vi "test_read-nmea-data2.vi"() -> ()   [LabVIEW 2019] (continued)
15:10:14.81\tF9P\t\t\n15:10:14.83\tF9P\t\t\n15:10:14.85\tF9P\t\t\n15:10:14.87\tF9P\t\t\n15:10:14.89\tF9P\t\t\n15:10:14.91\tF9P\t\t\n15:10:14.93\tF9P\t\t\n15:10:14.95\tF9P\t\t\n15:10:14.97\tF9P\t\t\n15:10:14.99\tF9P\t\t\n15:10:15.01\tF9P\t\t\n15:10:15.03\tF9P\t\t\n15:10:15.05\tF9P\t\t\n15:10:15.07\tF9P\t\t\n15:10:15.09\tF9P\t\t\n15:10:15.11\tF9P\t\t\n15:10:15.13\tF9P\t\t\n15:10:15.15\tF9P\t\t\n15:10:15.17\tF9P\t\t\n15:10:15.19\tF9P\t\t\n15:10:15.21\tF9P\t\t\n15:10:15.23\tF9P\t\t\n15:10:15.25\tF9P\t$GNRMC,061017.00,A,3723.57679,N,12656.88354,E,2.166,168.60,250720,,,A,V*08\n\t\n15:10:15.27\tF9P\t$GNVTG,168.60,T,,M,2.166,N,4.012,K,A*2E\n\t\n15:10:15.29\tF9P\t$GNGGA,061017.00,3723.57679,N,12656.88354,E,1,12,0.64,55.0,M,18.5,M,,*75\n\t\n15:10:15.31\tF9P\t$GNGSA,A,3,12,06,19,05,17,09,04,02,,,,,1.19,0.64,1.00,1*0A\n\t\n15:10:15.33\tF9P\t$GNGSA,A,3,85,71,84,,,,,,,,,,1.19,0.64,1.00,2*0F\n\t\n15:10:15.35\tF9P\t$GNGSA,A,3,36,19,11,04,09,12,,,,,,,1.19,0.64,1.00,3*0A\n\t\n15:10:15.37\tF9P\t$GNGSA,A,3,14,11,33,,,,,,,,,,1.19,0.64,1.00,4*0B\n\t\n15:10:15.39\tF9P\t$GPGSV,3,1,09,02,54,318,25,04,19,044,12,05,36,246,25,06,65,046,24,1*68\n\t\n15:10:15.41\tF9P\t$GPGSV,3,2,09,09,45,075,27,12,24,278,17,17,34,153,21,19,53,156,23,1*65\n\t\n15:10:15.43\tF9P\t$GPGSV,3,3,09,25,12,307,,1*5D\n\t\n15:10:15.45\tF9P\t$GPGSV,3,1,09,02,54,318,,04,19,044,,05,36,246,14,06,65,046,16,6*68\n\t\n15:10:15.47\tF9P\t$GPGSV,3,2,09,09,45,075,,12,24,278,,17,34,153,,19,53,156,,6*63\n\t\n15:10:15.49\tF9P\t$GPGSV,3,3,09,25,12,307,,6*5A\n\t\n15:10:15.51\tF9P\t$GLGSV,2,1,08,69,12,031,,70,72,041,,71,51,205,17,72,03,209,,1*74\n\t\n15:10:15.53\tF9P\t$GLGSV,2,2,08,77,01,326,,84,21,121,09,85,70,063,21,86,35,329,,1*7E\n\t\n15:10:15.55\tF9P\t$GLGSV,2,1,08,69,12,031,,70,72,041,,71,51,205,21,72,03,209,,3*73\n\t\n15:10:15.57\tF9P\t$GLGSV,2,2,08,77,01,326,,84,21,121,11,85,70,063,20,86,35,329,,3*74\n\t\n15:10:15.59\tF9P\t$GAGSV,2,1,08,02,09,298,09,04,66,119,25,09,31,193,16,11,71,357,23,7*72\n\t\n15:10:15.61\tF9P\t$GAGSV,2,2,08,12,40,102,15,19,27,045,14,25,09,249,,36,25,308,14,7*7F\n\t\n15:10:15.63\tF9P\t$GAGSV,2,1,08,02,09,298,,04,66,119,23,09,31,193,,11,71,357,19,2*76\n\t\n15:10:15.65\tF9P\t$GAGSV,2,2,08,12,40,102,,19,27,045,,25,09,249,,36,25,308,,2*7E\n\t\n15:10:15.67\tF9P\t$GBGSV,1,1,03,11,50,131,23,14,87,138,20,33,60,219,22,1*4C\n\t\n15:10:15.69\tF9P\t$GBGSV,1,1,03,11,50,131,31,14,87,138,21,33,60,219,,3*4C\n\t\n15:10:15.71\tF9P\t$GNGLL,3723.57679,N,12656.88354,E,061017.00,A,A*7D\n\t\n15:10:15.73\tF9P\t\t\n15:10:15.75\tF9P\t\t\n15:10:15.77\tF9P\t\t\n15:10:15.79\tF9P\t\t\n15:10:15.81\tF9P\t\t\n15:10:15.83\tF9P\t\t\n15:10:15.85\tF9P\t\t\n15:10:15.87\tF9P\t\t\n15:10:15.89\tF9P\t\t\n15:10:15.91\tF9P\t\t\n15:10:15.93\tF9P\t\t\n15:10:15.95\tF9P\t\t\n15:10:15.97\tF9P\t\t\n15:10:15.99\tF9P\t\t\n15:10:16.01\tF9P\t\t\n15:10:16.03\tF9P\t\t\n15:10:16.05\tF9P\t\t\n15:10:16.07\tF9P\t\t\n15:10:16.09\tF9P\t\t\n15:10:16.11\tF9P\t\t\n15:10:16.13\tF9P\t\t\n15:10:16.15\tF9P\t\t\n15:10:16.17\tF9P\t\t\n15:10:16.19\tF9P\t\t\n15:10:16.21\tF9P\t\t\n15:10:16.23\tF9P\t\t\n15:10:16.25\tF9P\t$GNRMC,061018.00,A,3723.57613,N,12656.88385,E,2.313,163.57,250720,,,A,V*08\n\t\n15:10:16.27\tF9P\t$GNVTG,163.57,T,,M,2.313,N,4.284,K,A*2C\n\t\n15:10:16.29\tF9P\t$GNGGA,061018.00,3723.57613,N,12656.88385,E,1,12,0.64,55.5,M,18.5,M,,*7F\n\t\n15:10:16.31\tF9P\t$GNGSA,A,3,12,06,19,05,17,09,04,02,,,,,1.19,0.64,1.00,1*0A\n\t\n15:10:16.33\tF9P\t$GNGSA,A,3,85,71,84,,,,,,,,,,1.19,0.64,1.00,2*0F\n\t\n15:10:16.36\tF9P\t$GNGSA,A,3,36,19,11,04,09,12,,,,,,,1.19,0.64,1.00,3*0A\n\t\n15:10:16.38\tF9P\t$GNGSA,A,3,14,11,33,,,,,,,,,,1.19,0.64,1.00,4*0B\n\t\n15:10:16.40\tF9P\t$GPGSV,3,1,09,02,54,318,25,04,19,044,13,05,36,246,24,06,65,046,25,1*69\n\t\n15:10:16.42\tF9P\t$GPGSV,3,2,09,09,45,075,32,12,24,278,17,17,34,153,23,19,53,156,23,1*63\n\t\n15:10:16.44\tF9P\t$GPGSV,3,3,09,25,12,307,,1*5D\n\t\n15:10:16.46\tF9P\t$GPGSV,3,1,09,02,54,318,,04,19,044,,05,36,246,15,06,65,046,15,6*6A\n\t\n15:10:16.48\tF9P\t$GPGSV,3,2,09,09,45,075,,12,24,278,,17,34,153,,19,53,156,,6*63\n\t\n15:10:16.50\tF9P\t$GPGSV,3,3,09,25,12,307,,6*5A\n\t\n15:10:16.52\tF9P\t$GLGSV,2,1,08,69,12,031,,70,72,041,,71,51,205,16,72,03,209,,1*75\n\t\n15:10:16.54\tF9P\t$GLGSV,2,2,08,77,01,326,,84,21,121,11,85,70,063,21,86,35,329,,1*77\n\t\n15:10:16.56\tF9P\t$GLGSV,2,1,08,69,12,031,,70,72,041,,71,51,205,21,72,03,209,,3*73\n\t\n15:10:16.58\tF9P\t$GLGSV,2,2,08,77,01,326,,84,21,121,09,85,70,063,20,86,35,329,,3*7D\n\t\n15:10:16.60\tF9P\t$GAGSV,2,1,08,02,09,298,10,04,66,119,23,09,31,193,16,11,71,357,24,7*7B\n\t\n15:10:16.62\tF9P\t$GAGSV,2,2,08,12,40,102,16,19,27,045,15,25,09,249,,36,25,308,12,7*7B\n\t\n15:10:16.64\tF9P\t$GAGSV,2,1,08,02,09,298,,04,66,119,,09,31,193,,11,71,357,17,2*79\n\t\n15:10:16.66\tF9P\t$GAGSV,2,2,08,12,40,102,,19,27,045,,25,09,249,,36,25,308,,2*7E\n\t\n15:10:16.68\tF9P\t$GBGSV,1,1,03,11,50,131,22,14,87,138,20,33,60,219,22,1*4D\n\t\n15:10:16.70\tF9P\t$GBGSV,1,1,03,11,50,131,,14,87,138,22,33,60,219,,3*4D\n\t\n15:10:16.72\tF9P\t$GNGLL,3723.57613,N,12656.88385,E,061018.00,A,A*72\n\t\n15:10:16.74\tF9P\t\t\n15:10:16.76\tF9P\t\t\n15:10:16.78\tF9P\t\t\n15:10:16.80\tF9P\t\t\n15:10:16.82\tF9P\t\t\n15:10:16.84\tF9P\t\t\n15:10:16.86\tF9P\t\t\n15:10:16.88\tF9P\t\t\n15:10:16.90\tF9P\t\t\n15:10:16.92\tF9P\t\t\n15:10:16.94\tF9P\t\t\n15:10:16.96\tF9P\t\t\n15:10:16.98\tF9P\t\t\n15:10:17.00\tF9P\t\t\n15:10:17.02\tF9P\t\t\n15:10:17.04\tF9P\t\t\n15:10:17.06\tF9P\t\t\n15:10:17.08\tF9P\t\t\n15:10:17.10\tF9P\t\t\n15:10:17.12\tF9P\t\t\n15:10:17.14\tF9P\t\t\n15:10:17.16\tF9P\t\t\n15:10:17.18\tF9P\t\t\n15:10:17.20\tF9P\t\t\n15:10:17.22\tF9P\t\t\n15:10:17.24\tF9P\t$GNRMC,061019.00,A,3723.57563,N,12656.88365,E,1.827,,250720,,,A,V*14\n\t\n15:10:17.26\tF9P\t$GNVTG,,T,,M,1.827,N,3.383,K,A*3A\n\t\n15:10:17.28\tF9P\t$GNGGA,061019.00,3723.57563,N,12656.88365,E,1,12,0.64,55.5,M,18.5,M,,*74\n\t\n15:10:17.30\tF9P\t$GNGSA,A,3,12,06,19,05,17,09,04,02,,,,,1.19,0.64,1.00,1*0A\n\t\n15:10:17.32\tF9P\t$GNGSA,A,3,85,71,84,,,,,,,,,,1.19,0.64,1.00,2*0F\n\t\n15:10:17.34\tF9P\t$GNGSA,A,3,36,19,11,04,09,12,,,,,,,1.19,0.64,1.00,3*0A\n\t\n15:10:17.36\tF9P\t$GNGSA,A,3,14,11,33,,,,,,,,,,1.19,0.64,1.00,4*0B\n\t\n15:10:17.38\tF9P\t$GPGSV,3,1,09,02,54,318,25,04,19,044,13,05,36,246,25,06,65,046,27,1*6A\n\t\n15:10:17.40\tF9P\t$GPGSV,3,2,09,09,45,075,31,12,24,278,17,17,34,153,22,19,53,156,23,1*61\n\t\n15:10:17.42\tF9P\t$GPGSV,3,3,09,25,12,307,17,1*5B\n\t\n15:10:17.44\tF9P\t$GPGSV,3,1,09,02,54,318,,04,19,044,,05,36,246,16,06,65,046,15,6*69\n\t\n15:10:17.46\tF9P\t$GPGSV,3,2,09,09,45,075,,12,24,278,,17,34,153,,19,53,156,,6*63\n\t\n15:10:17.48\tF9P\t$GPGSV,3,3,09,25,12,307,,6*5A\n\t\n15:10:17.50\tF9P\t$GLGSV,2,1,08,69,12,031,,70,72,041,,71,51,205,17,72,03,209,,1*74\n\t\n15:10:17.52\tF9P\t$GLGSV,2,2,08,77,01,326,,84,21,121,08,85,70,063,19,86,35,329,,1*74\n\t\n15:10:17.54\tF9P\t$GLGSV,2,1,08,69,12,031,,70,72,041,,71,51,205,20,72,03,209,,3*72\n\t\n15:10:17.56\tF9P\t$GLGSV,2,2,08,77,01,326,,84,21,121,11,85,70,063,19,86,35,329,,3*7E\n\t\n15:10:17.58\tF9P\t$GAGSV,2,1,08,02,09,298,12,04,66,119,22,09,31,193,17,11,71,357,23,7*7E\n\t\n15:10:17.60\tF9P\t$GAGSV,2,2,08,12,40,102,15,19,27,045,16,25,09,249,,36,25,308,13,7*7A\n\t\n15:10:17.62\tF9P\t$GAGSV,2,1,08,02,09,298,,04,66,119,,09,31,193,,11,71,357,14,2*7A\n\t\n15:10:17.64\tF9P\t$GAGSV,2,2,08,12,40,102,,19,27,045,,25,09,249,,36,25,308,,2*7E\n\t\n15:10:17.66\tF9P\t$GBGSV,1,1,03,11,50,131,21,14,87,138,19,33,60,219,21,1*47\n\t\n15:10:17.68\tF9P\t$GBGSV,1,1,03,11,50,131,,14,87,138,20,33,60,219,,3*4F\n\t\n15:10:17.70\tF9P\t$GNGLL,3723.57563,N,12656.88365,E,061019.00,A,A*79\n\t\n15:10:17.72\tF9P\t\t\n15:10:17.74\tF9P\t\t\n15:10:17.76\tF9P\t\t\n15:10:17.78\tF9P\t\t\n15:10:17.80\tF9P\t\t\n15:10:17.82\tF9P\t\t\n15:10:17.84\tF9P\t\t\n15:10:17.86\tF9P\t\t\n15:10:17.88\tF9P\t\t\n15:10:17.90\tF9P\t\t\n15:10:17.92\tF9P\t\t\n15:10:17.94\tF9P\t\t\n15:10:17.96\tF9P\t\t\n15:10:17.98\tF9P\t\t\n15:10:18.00\tF9P\t\t\n15:10:18.02\tF9P\t\t\n15:10:18.04\tF9P\t\t\n15:10:18.06\tF9P\t\t\n15:10:18.08\tF9P\t\t\n15:10:18.10\tF9P\t\t\n15:10:18.12\tF9P\t\t\n15:10:18.14\tF9P\t\t\n15:10:18.16\tF9P\t\t\n15:10:18.18\tF9P\t\t\n15:10:18.20\tF9P\t\t\n15:10:18.22\tF9P\t\t\n15:10:18.24\tF9P\t$GNRMC,061020.00,A,3723.57529,N,12656.88348,E,1.000,,250720,,,A,V*12\n\t\n15:10:18.26\tF9P\t$GNVTG,,T,,M,1.000,N,1.853,K,A*33\n\t\n15:10:18.28\tF9P\t$GNGGA,061020.00,3723.57529,N,12656.88348,E,1,12,0.64,56.6,M,18.5,M,,*7F\n\t\n15:10:18.30\tF9P\t$GNGSA,A,3,12,06,19,05,17,09,04,02,,,,,1.19,0.64,1.00,1*0A\n\t\n15:10:18.32\tF9P\t$GNGSA,A,3,85,71,84,,,,,,,,,,1.19,0.64,1.00,2*0F\n\t\n15:10:18.34\tF9P\t$GNGSA,A,3,36,19,11,04,09,12,,,,,,,1.19,0.64,1.00,3*0A\n\t\n15:10:18.36\tF9P\t$GNGSA,A,3,14,11,33,,,,,,,,,,1.19,0.64,1.00,4*0B\n\t\n15:10:18.38\tF9P\t$GPGSV,3,1,09,02,54,318,24,04,19,044,13,05,36,246,23,06,65,046,26,1*6C\n\t\n15:10:18.40\tF9P\t$GPGSV,3,2,09,09,45,075,30,12,24,278,17,17,34,153,22,19,53,156,24,1*67\n\t\n15:10:18.42\tF9P\t$GPGSV,3,3,09,25,12,307,15,1*59\n\t\n15:10:18.44\tF9P\t$GPGSV,3,1,09,02,54,318,,04,19,044,,05,36,246,15,06,65,046,15,6*6A\n\t\n15:10:18.46\tF9P\t$GPGSV,3,2,09,09,45,075,,12,24,278,,17,34,153,,19,53,156,,6*63\n\t\n15:10:18.48\tF9P\t$GPGSV,3,3,09,25,12,307,,6*5A\n\t\n15:10:18.50\tF9P\t$GLGSV,2,1,08,69,12,031,,70,72,041,,71,51,205,17,72,03,209,,1*74\n\t\n15:10:18.52\tF9P\t$GLGSV,2,2,08,77,01,326,,84,21,121,09,85,70,063,18,86,35,329,,1*74\n\t\n15:10:18.54\tF9P\t$GLGSV,2,1,08,69,12,031,,70,72,041,,71,51,205,20,72,03,209,,3*72\n\t\n15:10:18.56\tF9P\t$GLGSV,2,2,08,77,01,326,,84,21,121,08,85,70,063,19,86,35,329,,3*76\n\t\n15:10:18.58\tF9P\t$GAGSV,2,1,08,02,09,298,06,04,66,119,23,09,31,193,18,11,71,357,25,7*73\n\t\n15:10:18.60\tF9P\t$GAGSV,2,2,08,12,40,102,14,19,27,045,16,25,09,249,,36,25,308,14,7*7C\n\t\n15:10:18.62\tF9P\t$GAGSV,2,1,08,02,09,298,,04,66,119,,09,31,193,,11,71,357,14,2*7A\n\t\n15:10:18.64\tF9P\t$GAGSV,2,2,08,12,40,102,,19,27,045,,25,09,249,,36,25,308,,2*7E\n\t\n15:10:18.66\tF9P\t$GBGSV,1,1,03,11,50,131,21,14,87,138,19,33,60,219,21,1*47\n\t\n15:10:18.68\tF9P\t$GBGSV,1,1,03,11,50,131,,14,87,138,22,33,60,219,,3*4D\n\t\n15:10:18.70\tF9P\t$GNGLL,3723.57529,N,12656.88348,E,061020.00,A,A*72\n\t\n15:10:18.72\tF9P\t\t\n15:10:18.74\tF9P\t\t\n15:10:18.76\tF9P\t\t\n15:10:18.78\tF9P\t\t\n15:10:18.80\tF9P\t\t\n15:10:18.82\tF9P\t\t\n15:10:18.84\tF9P\t\t\n15:10:18.86\tF9P\t\t\n15:10:18.88\tF9P\t\t\n15:10:18.90\tF9P\t\t\n15:10:18.92\tF9P\t\t\n15:10:18.94\tF9P\t\t\n15:10:18.96\tF9P\t\t\n15:10:18.98\tF9P\t\t\n15:10:19.00\tF9P\t\t\n15:10:19.02\tF9P\t\t\n15:10:19.04\tF9P\t\t\n15:10:19.06\tF9P\t\t\n15:10:19.08\tF9P\t\t\n15:10:19.10\tF9P\t\t\n15:10:19.12\tF9P\t\t\n15:10:19.14\tF9P\t\t\n15:10:19.16\tF9P\t\t\n15:10:19.18\tF9P\t\t\n15:10:19.20\tF9P\t\t\n15:10:19.22\tF9P\t\t\n15:10:19.24\tF9P\t$GNRMC,061021.00,A,3723.57492,N,12656.88360,E,1.046,,250720,,,A,V*1A\n\t\n15:10:19.26\tF9P\t$GNVTG,,T,,M,1.046,N,1.938,K,A*3D\n\t\n15:10:19.28\tF9P\t$GNGGA,061021.00,3723.57492,N,12656.88360,E,1,12,0.64,57.4,M,18.5,M,,*76\n\t\n15:10:19.30\tF9P\t$GNGSA,A,3,12,06,19,05,17,09,04,02,,,,,1.19,0.64,1.00,1*0A\n\t\n15:10:19.32\tF9P\t$GNGSA,A,3,85,71,84,,,,,,,,,,1.19,0.64,1.00,2*0F\n\t\n15:10:19.34\tF9P\t$GNGSA,A,3,36,19,11,04,09,12,,,,,,,1.19,0.64,1.00,3*0A\n\t\n15:10:19.36\tF9P\t$GNGSA,A,3,14,11,33,,,,,,,,,,1.19,0.64,1.00,4*0B\n\t\n15:10:19.38\tF9P\t$GPGSV,3,1,09,02,54,318,24,04,19,044,12,05,36,246,28,06,65,046,25,1*65\n\t\n15:10:19.40\tF9P\t$GPGSV,3,2,09,09,45,075,23,12,24,278,18,17,34,153,22,19,53,156,25,1*6B\n\t\n15:10:19.42\tF9P\t$GPGSV,3,3,09,25,12,307,14,1*58\n\t\n15:10:19.44\tF9P\t$GPGSV,3,1,09,02,54,318,,04,19,044,,05,36,246,15,06,65,046,14,6*6B\n\t\n15:10:19.46\tF9P\t$GPGSV,3,2,09,09,45,075,,12,24,278,,17,34,153,,19,53,156,,6*63\n\t\n15:10:19.48\tF9P\t$GPGSV,3,3,09,25,12,307,,6*5A\n\t\n15:10:19.50\tF9P\t$GLGSV,2,1,08,69,12,031,,70,72,041,,71,51,205,19,72,03,209,,1*7A\n\t\n15:10:19.52\tF9P\t$GLGSV,2,2,08,77,01,326,,84,20,122,11,85,70,063,20,86,35,329,,1*74\n\t\n15:10:19.54\tF9P\t$GLGSV,2,1,08,69,12,031,,70,72,041,,71,51,205,20,72,03,209,,3*72\n\t\n15:10:19.56\tF9P\t$GLGSV,2,2,08,77,01,326,,84,20,122,10,85,70,063,18,86,35,329,,3*7C\n\t\n15:10:19.58\tF9P\t$GAGSV,2,1,08,02,09,298,09,04,66,119,23,09,31,193,18,11,71,357,24,7*7D\n\t\n15:10:19.60\tF9P\t$GAGSV,2,2,08,12,40,102,14,19,27,045,16,25,09,249,,36,25,308,14,7*7C\n\t\n15:10:19.62\tF9P\t$GAGSV,2,1,08,02,09,298,,04,66,119,,09,31,193,27,11,71,357,15,2*7E\n\t\n15:10:19.64\tF9P\t$GAGSV,2,2,08,12,40,102,,19,27,045,,25,09,249,,36,25,308,,2*7E\n\t\n15:10:19.66\tF9P\t$GBGSV,1,1,03,11,50,131,20,14,87,138,19,33,60,219,21,1*46\n\t\n15:10:19.68\tF9P\t$GBGSV,1,1,03,11,50,131,,14,87,138,22,33,60,219,,3*4D\n\t\n15:10:19.70\tF9P\t$GNGLL,3723.57492,N,12656.88360,E,061021.00,A,A*78\n\t\n15:10:19.72\tF9P\t\t\n15:10:19.74\tF9P\t\t\n15:10:19.76\tF9P\t\t\n15:10:19.78\tF9P\t\t\n15:10:19.80\tF9P\t\t\n15:10:19.82\tF9P\t\t\n15:10:19.84\tF9P\t\t\n15:10:19.86\tF9P\t\t\n15:10:19.88\tF9P\t\t\n15:10:19.90\tF9P\t\t\n15:10:19.92\tF9P\t\t\n15:10:19.94\tF9P\t\t\n15:10:19.96\tF9P\t\t\n15:10:19.98\tF9P\t\t\n15:10:20.00\tF9P\t\t\n15:10:20.02\tF9P\t\t\n15:10:20.04\tF9P\t\t\n15:10:20.06\tF9P\t\t\n15:10:20.08\tF9P\t\t\n15:10:20.10\tF9P\t\t\n15:10:20.12\tF9P\t\t\n15:10:20.14\tF9P\t\t\n15:10:20.16\tF9P\t\t\n15:10:20.18\tF9P\t\t\n15:10:20.20\tF9P\t\t\n15:10:20.22\tF9P\t\t\n15:10:20.24\tF9P\t$GNRMC,061022.00,A,3723.57424,N,12656.88360,E,1.903,,250720,,,A,V*1C\n\t\n15:10:20.26\tF9P\t$GNVTG,,T,,M,1.903,N,3.524,K,A*36\n\t\n15:10:20.28\tF9P\t$GNGGA,061022.00,3723.57424,N,12656.88360,E,1,12,0.64,57.6,M,18.5,M,,*7A\n\t\n15:10:20.30\tF9P\t$GNGSA,A,3,12,06,19,05,17,09,04,02,,,,,1.19,0.64,1.00,1*0A\n\t\n15:10:20.32\tF9P\t$GNGSA,A,3,85,71,84,,,,,,,,,,1.19,0.64,1.00,2*0F\n\t\n15:10:20.34\tF9P\t$GNGSA,A,3,36,19,11,04,09,12,,,,,,,1.19,0.64,1.00,3*0A\n\t\n15:10:20.36\tF9P\t$GNGSA,A,3,14,11,33,,,,,,,,,,1.19,0.64,1.00,4*0B\n\t\n15:10:20.38\tF9P\t$GPGSV,3,1,09,02,54,318,24,04,19,044,12,05,36,246,24,06,65,046,31,1*6C\n\t\n15:10:20.40\tF9P\t$GPGSV,3,2,09,09,45,075,30,12,24,278,19,17,34,153,23,19,53,156,22,1*6E\n\t\n15:10:20.42\tF9P\t$GPGSV,3,3,09,25,12,307,14,1*58\n\t\n15:10:20.44\tF9P\t$GPGSV,3,1,09,02,54,318,,04,19,044,,05,36,246,16,06,65,046,13,6*6F\n\t\n15:10:20.46\tF9P\t$GPGSV,3,2,09,09,45,075,,12,24,278,,17,34,153,,19,53,156,,6*63\n\t\n15:10:20.48\tF9P\t$GPGSV,3,3,09,25,12,307,,6*5A\n\t\n15:10:20.50\tF9P\t$GLGSV,2,1,08,69,12,031,,70,72,041,,71,51,205,20,72,03,209,,1*70\n\t\n15:10:20.52\tF9P\t$GLGSV,2,2,08,77,01,326,,84,20,122,08,85,70,065,20,86,35,329,,1*7A\n\t\n15:10:20.54\tF9P\t$GLGSV,2,1,08,69,12,031,,70,72,041,,71,51,205,20,72,03,209,,3*72\n\t\n15:10:20.56\tF9P\t$GLGSV,2,2,08,77,01,326,,84,20,122,08,85,70,065,19,86,35,329,,3*72\n\t\n15:10:20.58\tF9P\t$GAGSV,2,1,08,02,09,298,08,04,66,119,22,09,31,193,17,11,71,357,24,7*72\n\t\n15:10:20.60\tF9P\t$GAGSV,2,2,08,12,40,102,12,19,27,045,15,25,09,249,,36,25,308,15,7*78\n\t\n15:10:20.62\tF9P\t$GAGSV,2,1,08,02,09,298,,04,66,119,,09,31,193,24,11,71,357,15,2*7D\n\t\n15:10:20.64\tF9P\t$GAGSV,2,2,08,12,40,102,,19,27,045,,25,09,249,,36,25,308,,2*7E\n\t\n15:10:20.66\tF9P\t$GBGSV,1,1,03,11,50,131,20,14,87,138,20,33,60,219,21,1*4C\n\t\n15:10:20.68\tF9P\t$GBGSV,1,1,03,11,50,131,,14,87,138,22,33,60,219,,3*4D\n\t\n15:10:20.70\tF9P\t$GNGLL,3723.57424,N,12656.88360,E,061022.00,A,A*76\n\t\n15:10:20.72\tF9P\t\t\n15:10:20.74\tF9P\t\t\n15:10:20.76\tF9P\t\t\n15:10:20.78\tF9P\t\t\n15:10:20.80\tF9P\t\t\n15:10:20.82\tF9P\t\t\n15:10:20.84\tF9P\t\t\n15:10:20.86\tF9P\t\t\n15:10:20.88\tF9P\t\t\n15:10:20.91\tF9P\t\t\n15:10:20.93\tF9P\t\t\n15:10:20.95\tF9P\t\t\n15:10:20.97\tF9P\t\t\n15:10:20.99\tF9P\t\t\n15:10:21.01\tF9P\t\t\n15:10:21.03\tF9P\t\t\n15:10:21.05\tF9P\t\t\n15:10:21.07\tF9P\t\t\n15:10:21.09\tF9P\t\t\n15:10:21.11\tF9P\t\t\n15:10:21.12\tF9P\t\t\n15:10:21.14\tF9P\t\t\n15:10:21.16\tF9P\t\t\n15:10:21.18\tF9P\t\t\n15:10:21.20\tF9P\t\t\n15:10:21.22\tF9P\t\t\n15:10:21.24\tF9P\t$GNRMC,061023.00,A,3723.57354,N,12656.88377,E,1.992,,250720,,,A,V*13\n\t\n15:10:21.26\tF9P\t$GNVTG,,T,,M,1.992,N,3.689,K,A*3A\n\t\n15:10:21.28\tF9P\t$GNGGA,061023.00,3723.57354,N,12656.88377,E,1,12,0.64,58.0,M,18.5,M,,*74\n\t\n15:10:21.30\tF9P\t$GNGSA,A,3,12,06,19,05,17,09,04,02,,,,,1.19,0.64,1.00,1*0A\n\t\n15:10:21.32\tF9P\t$GNGSA,A,3,85,71,84,,,,,,,,,,1.19,0.64,1.00,2*0F\n\t\n15:10:21.34\tF9P\t$GNGSA,A,3,36,19,11,04,09,12,,,,,,,1.19,0.64,1.00,3*0A\n\t\n15:10:21.36\tF9P\t$GNGSA,A,3,14,11,33,,,,,,,,,,1.19,0.64,1.00,4*0B\n\t\n15:10:21.38\tF9P\t$GPGSV,3,1,09,02,54,318,23,04,19,044,12,05,36,246,24,06,65,046,25,1*6E\n\t\n15:10:21.40\tF9P\t$GPGSV,3,2,09,09,45,075,24,12,24,278,18,17,34,153,22,19,53,156,22,1*6B\n\t\n15:10:21.42\tF9P\t$GPGSV,3,3,09,25,12,307,15,1*59\n\t\n15:10:21.44\tF9P\t$GPGSV,3,1,09,02,54,318,,04,19,044,,05,36,246,17,06,65,046,12,6*6F\n\t\n15:10:21.46\tF9P\t$GPGSV,3,2,09,09,45,075,,12,24,278,,17,34,153,,19,53,156,,6*63\n\t\n15:10:21.48\tF9P\t$GPGSV,3,3,09,25,12,307,,6*5A\n\t\n15:10:21.50\tF9P\t$GLGSV,2,1,08,69,12,031,,70,72,041,,71,51,205,19,72,03,209,,1*7A\n\t\n15:10:21.52\tF9P\t$GLGSV,2,2,08,77,01,326,,84,20,122,08,85,70,065,21,86,36,330,,1*70\n\t\n15:10:21.54\tF9P\t$GLGSV,2,1,08,69,12,031,,70,72,041,,71,51,205,20,72,03,209,,3*72\n\t\n15:10:21.56\tF9P\t$GLGSV,2,2,08,77,01,326,,84,20,122,10,85,70,065,19,86,36,330,,3*70\n\t\n15:10:21.58\tF9P\t$GAGSV,2,1,08,02,09,298,08,04,66,119,22,09,31,193,17,11,71,357,24,7*72\n\t\n15:10:21.60\tF9P\t$GAGSV,2,2,08,12,40,102,10,19,27,045,18,25,09,249,,36,25,308,14,7*76\n\t\n15:10:21.62\tF9P\t$GAGSV,2,1,08,02,09,298,,04,66,119,,09,31,193,21,11,71,357,12,2*7F\n\t\n15:10:21.64\tF9P\t$GAGSV,2,2,08,12,40,102,,19,27,045,,25,09,249,,36,25,308,,2*7E\n\t\n15:10:21.66\tF9P\t$GBGSV,1,1,03,11,50,131,21,14,87,138,20,33,60,219,21,1*4D\n\t\n15:10:21.68\tF9P\t$GBGSV,1,1,03,11,50,131,,14,87,138,21,33,60,219,,3*4E\n\t\n15:10:21.70\tF9P\t$GNGLL,3723.57354,N,12656.88377,E,061023.00,A,A*71\n\t\n15:10:21.72\tF9P\t\t\n15:10:21.74\tF9P\t\t\n15:10:21.76\tF9P\t\t\n15:10:21.78\tF9P\t\t\n15:10:21.80\tF9P\t\t\n15:10:21.82\tF9P\t\t\n15:10:21.84\tF9P\t\t\n15:10:21.86\tF9P\t\t\n15:10:21.88\tF9P\t\t\n15:10:21.90\tF9P\t\t\n15:10:21.92\tF9P\t\t\n15:10:21.94\tF9P\t\t\n15:10:21.96\tF9P\t\t\n15:10:21.98\tF9P\t\t\n15:10:22.00\tF9P\t\t\n15:10:22.02\tF9P\t\t\n15:10:22.04\tF9P\t\t\n15:10:22.06\tF9P\t\t\n15:10:22.08\tF9P\t\t\n15:10:22.10\tF9P\t\t\n15:10:22.12\tF9P\t\t\n15:10:22.14\tF9P\t\t\n15:10:22.16\tF9P\t\t\n15:10:22.18\tF9P\t\t\n15:10:22.20\tF9P\t\t\n15:10:22.22\tF9P\t\t\n15:10:22.24\tF9P\t$GNRMC,061024.00,A,3723.57293,N,12656.88370,E,1.879,,250720,,,A,V*1D\n\t\n15:10:22.26\tF9P\t$GNVTG,,T,,M,1.879,N,3.480,K,A*35\n\t\n15:10:22.28\tF9P\t$GNGGA,061024.00,3723.57293,N,12656.88370,E,1,12,0.65,59.5,M,18.5,M,,*7B\n\t\n15:10:22.30\tF9P\t$GNGSA,A,3,12,06,19,05,17,09,04,02,,,,,1.19,0.65,1.00,1*0B\n\t\n15:10:22.32\tF9P\t$GNGSA,A,3,85,71,84,,,,,,,,,,1.19,0.65,1.00,2*0E\n\t\n15:10:22.34\tF9P\t$GNGSA,A,3,36,19,11,04,09,,,,,,,,1.19,0.65,1.00,3*08\n\t\n15:10:22.36\tF9P\t$GNGSA,A,3,14,11,33,,,,,,,,,,1.19,0.65,1.00,4*0A\n\t\n15:10:22.38\tF9P\t$GPGSV,3,1,09,02,54,318,22,04,19,044,13,05,36,246,25,06,65,046,25,1*6F\n\t\n15:10:22.40\tF9P\t$GPGSV,3,2,09,09,45,075,25,12,24,278,18,17,34,153,22,19,53,156,22,1*6A\n\t\n15:10:22.42\tF9P\t$GPGSV,3,3,09,25,12,307,13,1*5F\n\t\n15:10:22.44\tF9P\t$GPGSV,3,1,09,02,54,318,,04,19,044,,05,36,246,18,06,65,046,15,6*67\n\t\n15:10:22.46\tF9P\t$GPGSV,3,2,09,09,45,075,,12,24,278,,17,34,153,,19,53,156,,6*63\n\t\n15:10:22.48\tF9P\t$GPGSV,3,3,09,25,12,307,,6*5A\n\t\n15:10:22.50\tF9P\t$GLGSV,2,1,08,69,12,031,,70,72,041,,71,51,205,18,72,03,209,,1*7B\n\t\n15:10:22.52\tF9P\t$GLGSV,2,2,08,77,01,326,,84,20,122,11,85,70,065,20,86,36,330,,1*79\n\t\n15:10:22.54\tF9P\t$GLGSV,2,1,08,69,12,031,,70,72,041,,71,51,205,20,72,03,209,,3*72\n\t\n15:10:22.56\tF9P\t$GLGSV,2,2,08,77,01,326,,84,20,122,13,85,70,065,20,86,36,330,,3*79\n\t\n15:10:22.58\tF9P\t$GAGSV,2,1,08,02,09,298,08,04,66,119,24,09,31,193,17,11,71,357,25,7*75\n\t\n15:10:22.60\tF9P\t$GAGSV,2,2,08,12,40,102,09,19,27,045,20,25,09,249,,36,25,308,14,7*75\n\t\n15:10:22.62\tF9P\t$GAGSV,2,1,08,02,09,298,,04,66,119,,09,31,193,20,11,71,357,10,2*7C\n\t\n15:10:22.64\tF9P\t$GAGSV,2,2,08,12,40,102,,19,27,045,,25,09,249,,36,25,
